vi "WLAN - niVST - OPPO - RFSG - Loadwaveform and Download.vi"(0 "instrument handle":refnum<k15>, 2 "ScriptName<index>":string="WLANRxTesting", 5 "file path":path, 9 "Idle Time (With Ack)":dbl, 11 "error in":errorcluster, 13 "numPackets":i32=100) -> (4 "instrument handle":refnum<k15>, 6 "Rx_Test Parameters":T1 {"OFDM Data Rate (Mbps)" items=["6", "9", "12", "18", "24", "36", "48", "54"]; "DSSS Data Rate (Mbps)" items=["1", "2", "5.5 CCK", "5.5 PBCC", "11 CCK", "11 PBCC", "22", "33"]; "80211n PLCP Frame Format" items=["Mixed Format", "Greenfield Format"]}, 15 "error out":errorcluster)   [LabVIEW 2012]
uses:
  TV/RW/Includes/WLAN - TV - RW - INC - RxTestParameters.ctl
  <instrlib>/niRFSG/niRFSG.llb/niRFSG Write Arb Waveform (Complex Input).vi
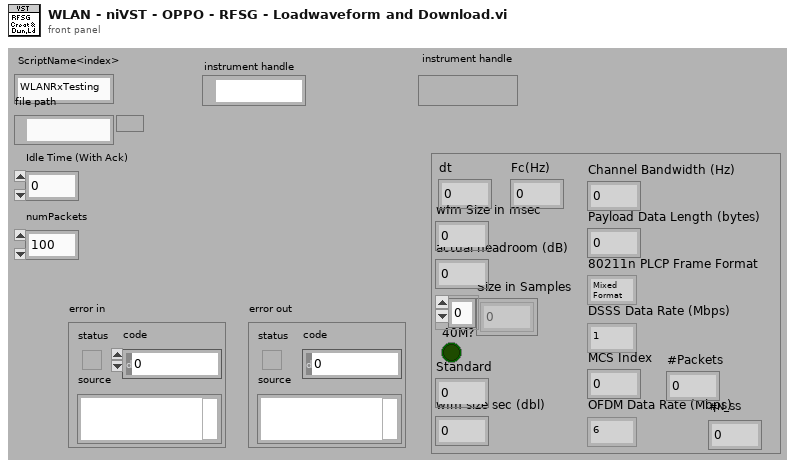
[diagram p1: front panel]
types:
  T1 = typedef "WLAN - TV - RW - INC - RxTestParameters.ctl" = cluster{"wfm Size in msec":i32, "actual headroom (dB)":dbl, "Size in Samples":i32[], "40M?":bool, "Standard ":i32, "wfm size sec (dbl)":dbl, "dt":dbl, "Channel Bandwidth (Hz)":dbl, "Payload Data Length (bytes)":i32, "80211n PLCP Frame Format":i32, "DSSS Data Rate (Mbps)":i32, "OFDM Data Rate (Mbps)":i32, "MCS Index":i32, "Fc(Hz)":dbl, "#Packets":i32, "#N_SS":i32}
  T2 = cluster{"Waveforms":cluster{"t0":dbl, "dt":dbl, "Y":cdb[]}[], "wfm Size in msec":i32, "actual headroom (dB)":dbl, "Size in Samples":i32[], "40M?":bool, "Standard ":i32, "wfm size sec (dbl)":dbl}
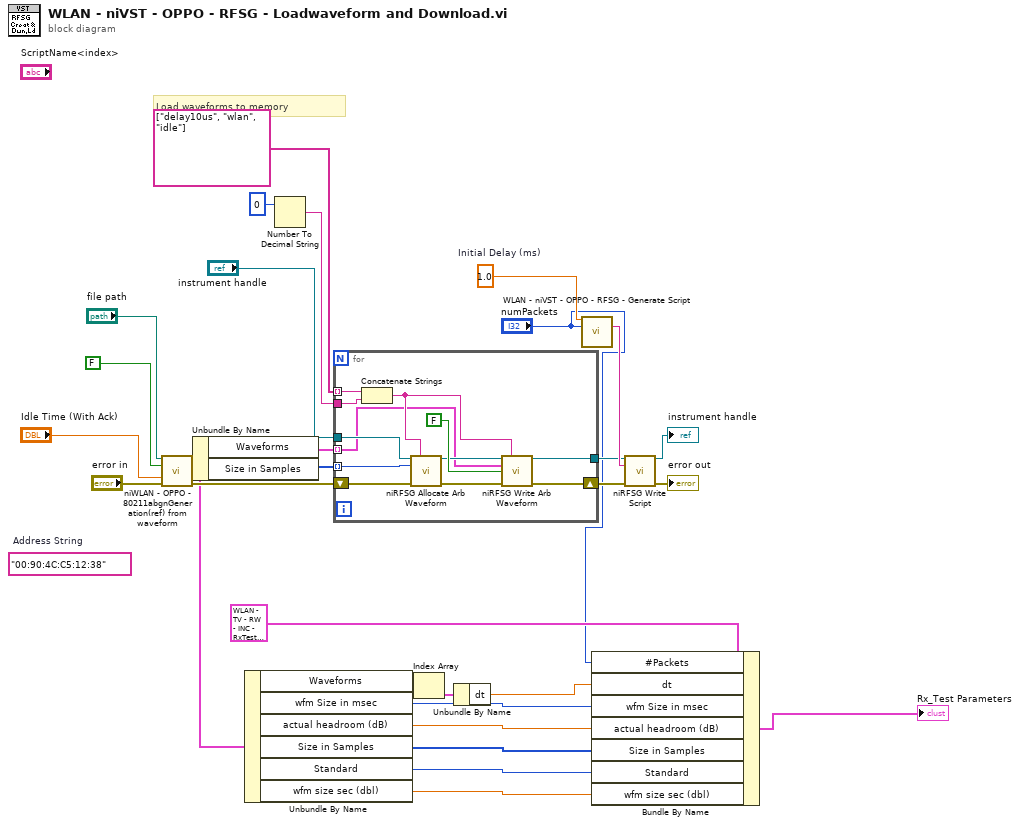
[diagram p0: block diagram]
diagram:
  (unwired) "00:90:4C:C5:12:38"  # Address String
  w29 = 1.0  # Initial Delay (ms)
  # "Load waveforms to memory"
  n1 = call "niWLAN - OPPO - 80211abgnGeneration(ref) from waveform.vi"("file path"="file path", "Without ACK ?"=FALSE ("w/ ACK"), "Idle Time (With Ack)"="Idle Time (With Ack)", "error in"="error in") -> ("Cluster"=w10:T2, "error out"=w24:errorcluster)  [unwired: 10 in]
  n2 = Unbundle By Name(w10) -> ("Waveforms"=w12:cluster{"t0":dbl, "dt":dbl, "Y":cdb[]}[], "Size in Samples"=w20:i32[])
  n3 = Unbundle By Name(w10) -> ("Waveforms"=w9:cluster{"t0":dbl, "dt":dbl, "Y":cdb[]}[], "wfm Size in msec"=w6:i32, "actual headroom (dB)"=w3:dbl, "Size in Samples"=w4:i32[], "Standard"=w5:i32, "wfm size sec (dbl)"=w2:dbl)
  n4 = Number To Decimal String(number=0) -> (decimal integer string=w19:string)  [unwired: 1 in]
  n5 = for {
    tunnel: [w38] -> w18
    tunnel: "instrument handle" -> [w35]
    shift-right: [w37] -> w17
    shift-left: w24 -> [w36]
    tunnel: string[] ["delay10us", "wlan", "idle"] -> [w33] mode=indexing
    tunnel: w20 -> [w34] mode=indexing
    tunnel: w12 -> [w30] mode=indexing
    tunnel: w19 -> [w32]
    n6 = Concatenate Strings(w33, w32) -> (w31:string)
    n7 = call <instrlib>:"niRFSG Allocate Arb Waveform.vi"("instrument handle"=w35, "name"=w31, "size in samples"=w34, "error in"=w36) -> ("instrument handle out"=w40:refnum<k15>, "error out"=w39:errorcluster)  [unwired: 10 in]
    n8 = call-poly <instrlib>:"niRFSG Write Arb Waveform.vi"("instrument handle"=w40, "name"=w31, "IQ waveform"=w30, "use waveform dt for IQ rate?"=FALSE, "error in"=w39) -> ("instrument handle out"=w38:refnum<k15>, "error out"=w37:errorcluster)  [unwired: 9 in]
  }
  n9 = Index Array(array=w9) -> (element=w8:cluster{"t0":dbl, "dt":dbl, "Y":cdb[]})  [unwired: 1 in]
  n10 = Unbundle By Name(w8) -> ("dt"=w7:dbl)
  n11 = call "WLAN - niVST - OPPO - RFSG - Generate Script.vi"("Initial Delay (ms)"=w29, "Number of Packets"="numPackets") -> ("resulting script"=w28:string)  [unwired: 13 in]
  n12 = Bundle By Name(cluster=T1 {"wfm Size in msec"=0, "actual headroom (dB)"=0.0, "Size in Samples"=[], "40M?"=FALSE, "Standard "=0, "wfm size sec (dbl)"=0.0, "dt"=0.0, "Channel Bandwidth (Hz)"=0.0, "Payload Data Length (bytes)"=0, "80211n PLCP Frame Format"=0, "DSSS Data Rate (Mbps)"=0, "OFDM Data Rate (Mbps)"=0, "MCS Index"=0, "Fc(Hz)"=0.0, "#Packets"=0, "#N_SS"=0} ("Cluster"), "#Packets"="numPackets", "dt"=w7, "wfm Size in msec"=w6, "actual headroom (dB)"=w3, "Size in Samples"=w4, "Standard"=w5, "wfm size sec (dbl)"=w2) -> (→"Rx_Test Parameters":T1)
  n13 = call <instrlib>:"niRFSG Write Script.vi"("instrument handle"=w18, "script"=w28, "error in"=w17) -> ("instrument handle out"=→"instrument handle":refnum<k15>, "error out"=→"error out":errorcluster)  [unwired: 11 in]
